vi "AddParametersToCMD.vi"(8 "error in (no error)":errorcluster, 10 "DynamicParameters in":refnum<class "DynamicParameters.lvclass">, 11 "CreateCommand":refnum<k24>) -> (0 "error out":errorcluster, 3 "CreateCommand Out":refnum<k24>)   [LabVIEW 2020, in "ORM_ADONet.lvlib" / "ADOMapper.lvclass"]
uses:
  ADOMapper.lvclass
  System.Data
  <vilib>/Viviota/shared/ORM.lvlibp/ORM/DynamicParameters/DynamicParameters.lvclass
  ADOParameter/ADOParameter.lvclass
  C:/Viviota/Projects/R&D/__OpenSource/VIV_ORM/libraries/npgsql/System.Text.Json.dll
  libraries/npgsql/System.Text.Json.dll
  <userlib>/_OpenG.lib/lvdata/lvdata.llb/openg_variant.lvlib
panel:
  out "error out 5":errorcluster
  out "error out 4":errorcluster
  out "error out 3":errorcluster
  out "error out 2":errorcluster
  out "DbType":i32[](array[ring]) items=["AnsiString"=0, "Binary"=1, "Byte"=2, "Boolean"=3, "Currency"=4, "Date"=5, "DateTime"=6, "Decimal"=7, "Double"=8, "Guid"=9, "Int16"=10, "Int32"=11, "Int64"=12, "Object"=13, "SByte"=14, "Single"=15, "String"=16, "Time"=17, "UInt16"=18, "UInt32"=19, "UInt64"=20, "VarNumeric"=21, "AnsiStringFixedLength"=22, "StringFixedLength"=23, "Xml"=25, "DateTime2"=26, "DateTimeOffset"=27]
  out "Array 2":string[](array[string])
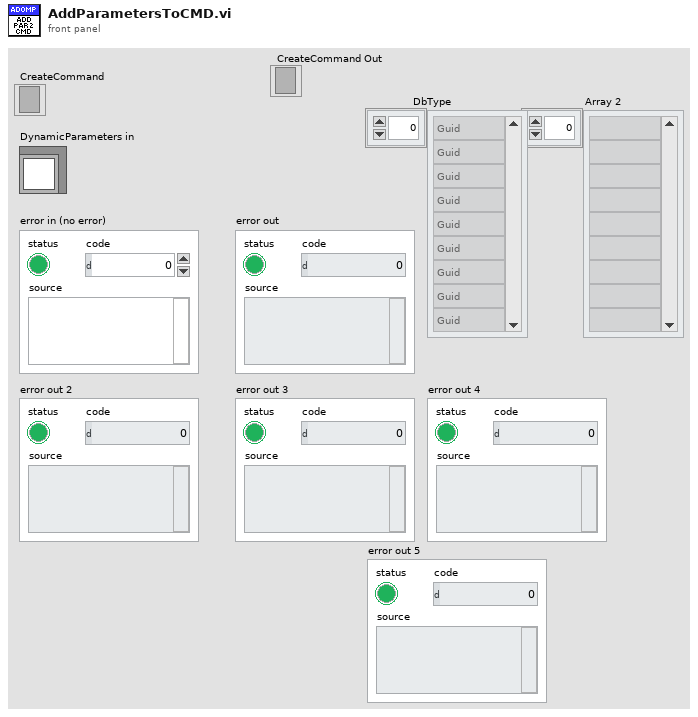
[diagram p1: front panel]
types:
  T1 = cluster{"DbType":i32, "Direction":i32, "Size":i32, "Precision":u8, "Scale":u8}[]
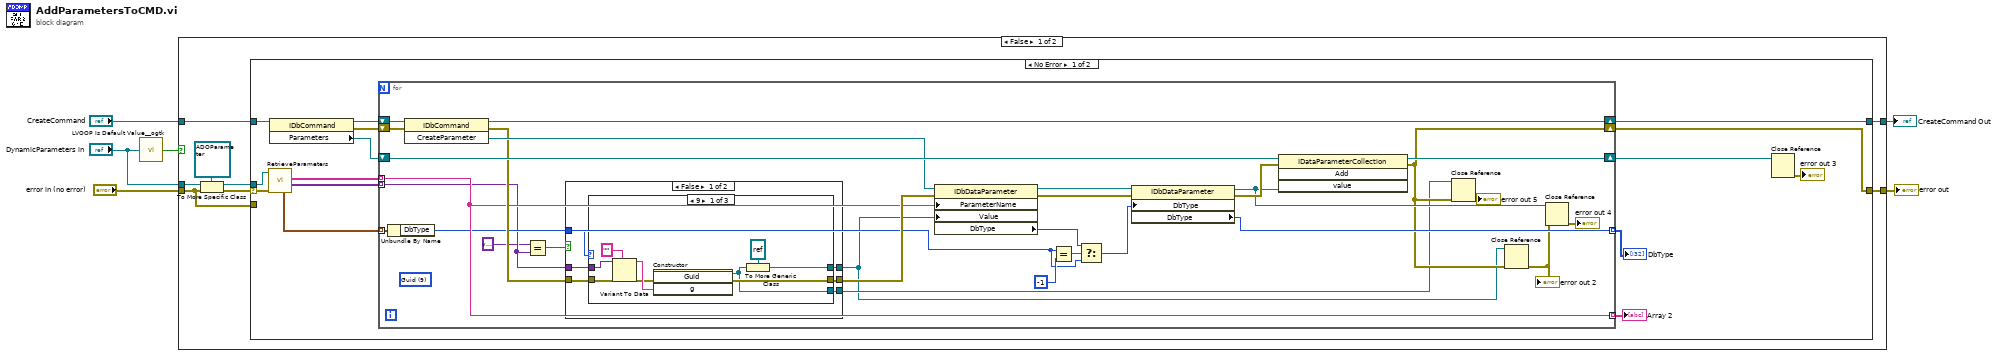
[diagram p0: block diagram]
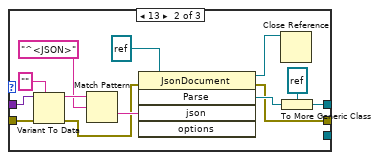
[diagram p2: hidden frame]
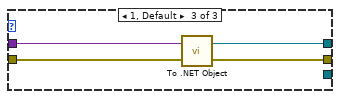
[diagram p3: hidden frame]
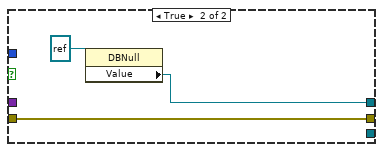
[diagram p4: hidden frame]
diagram:
  n1 = call <userlib>:"LVOOP Is Default Value__ogtk.vi"("Object"="DynamicParameters in") -> ("Is Default Value?"=w3:bool)
  n2 = case shown="False" w3 {
    tunnel: "error in (no error)" -> [w11 w97]
    tunnel: [w7 w97] -> w6
    tunnel: "DynamicParameters in" -> [w13 _]
    tunnel: "CreateCommand" -> [w9 w96]
    tunnel: [w8 w96] -> w1
    frame False {
      n3 = To More Specific Class(target class=refnum<class "ADOParameter.lvclass"> refnum ("ADONet.lvlib:ADOParameter.lvclass"), reference=w13, error in=w11) -> (specific class reference=w10:refnum<class "ADOParameter.lvclass">, error out=w12:errorcluster)
      n4 = case shown="No Error" w12 {
        selector: w12 -> [w29 w94]
        tunnel: w11 -> [_ _]
        tunnel: w10 -> [w28 _]
        tunnel: w9 -> [w27 w95]
        tunnel: [w21 w95] -> w8
        tunnel: [w20 w94] -> w7
        frame No Error {
          n5 = call "RetrieveParameters.vi"("error in (no error)"=w29, "ADOParameter in"=w28) -> ("Values"=w23:variant[], "Names"=w24:string[], "Options"=w18:T1)  [unwired: 5 in, 2 out]
          n6 = property class="IDbCommand"(reference=w27) -> (reference out=w26:refnum<k24>, error out=w22:errorcluster, "Parameters"=w25:refnum<k24>)  [unwired: 1 in]
          n7 = for {
            shift-right: [w51] -> w21
            shift-left: w26 -> [w58]
            shift-right: [w56] -> w15
            shift-left: w25 -> [w57]
            tunnel: w24 -> [w50] mode=indexing
            tunnel: w23 -> [w40] mode=indexing
            shift-right: [w33] -> w20
            shift-left: w22 -> [w52]
            tunnel: [w43] -> w17 mode=indexing
            tunnel: [w50] -> w19 mode=indexing
            tunnel: w18 -> [w42] mode=indexing
            (unwired) 9 items=["AnsiString"=0, "Binary"=1, "Byte"=2, "Boolean"=3, "Currency"=4, "Date"=5, "DateTime"=6, "Decimal"=7, "Double"=8, "Guid"=9, "Int16"=10, "Int32"=11, "Int64"=12, "Object"=13, "SByte"=14, "Single"=15, "String"=16, "Time"=17, "UInt16"=18, "UInt32"=19, "UInt64"=20, "VarNumeric"=21, "AnsiStringFixedLength"=22, "StringFixedLength"=23, "Xml"=25, "DateTime2"=26, "DateTimeOffset"=27] ("DbType")
            n8 = Unbundle By Name(w42) -> ("DbType"=w41:i32)
            n9 = invoke class="IDbCommand" method="CreateParameter"(reference=w58, error in=w52) -> (reference out=w51:refnum<k24>, error out=w54:errorcluster, "CreateParameter"=w55:refnum<k24>)  [unwired: 1 in]
            n10 = Equal?(x=variant, y=w40) -> (x = y?=w37:bool)
            n11 = case shown="False" w37 {
              tunnel: w54 -> [w64 w93]
              tunnel: [w63 w93] -> w53
              tunnel: w41 -> [w62 _]
              tunnel: [w61 w91] -> w30
              tunnel: w40 -> [w60 _]
              tunnel: [w59 _] -> w32
              frame False {
                n12 = case shown="9" w62 {
                  tunnel: [w67 w74 w87] -> w61
                  tunnel: w64 -> [w73 w75 w90]
                  tunnel: [w68 w78 w89] -> w63
                  tunnel: w60 -> [w72 w76 w88]
                  tunnel: [w65 _ _] -> w59
                  frame 9 {
                    n13 = Variant To Data(error in=w73, type="", Variant=w72) -> (data=w70:string, error out=w69:errorcluster)
                    n14 = constructor class="System.Guid" ("Constructor Node")(error in=w69, "g"=w70) -> (reference out=w65:refnum<k24>, error out=w68:errorcluster)  [unwired: 2 in, 2 out]
                    n15 = To More Generic Class(target class=refnum<k24> refnum ("Value"), reference=w65) -> (generic class reference=w67:refnum<k24>)
                  }
                  frame 13 {
                    n16 = Variant To Data(error in=w75, type="", Variant=w76) -> (data=w85:string, error out=w81:errorcluster)
                    n17 = Match Pattern(string=w85, regular expression="^<JSON>") -> (after substring=w82:string)  [unwired: 1 in, 3 out]
                    n18 = invoke class="JsonDocument" method="Parse"(reference=refnum<k24> refnum ("Value"), error in=w81, "json"=w82) -> (reference out=w79:refnum<k24>, error out=w78:errorcluster, "Parse"=w80:refnum<k24>)  [unwired: 2 in, 2 out]
                    n19 = Close Reference(reference=w79) -> ()  [unwired: 1 in, 1 out]
                    n20 = To More Generic Class(target class=refnum<k24> refnum ("Value"), reference=w80) -> (generic class reference=w74:refnum<k24>)
                  }
                  frame 1, Default {
                    n21 = call <vilib>:"To .NET Object.vi"("error in (no error)"=w90, "anything"=w88) -> ("error out"=w89:errorcluster, ".NET object"=w87:refnum<k24>)
                  }
                }
              }
              frame True {
                n22 = property class="DBNull"(reference=refnum<k24> refnum ("CreateParameter")) -> ("Value"=w91:refnum<k24>)  [unwired: 1 in, 2 out]
              }
            }
            n23 = property class="IDbDataParameter"(reference=w55, error in=w53, "ParameterName"=w50, "Value"=w30) -> (reference out=w49:refnum<k24>, error out=w47:errorcluster, "DbType"=w38:i32)
            n24 = Equal?(x=w41, y=-1) -> (x = y?=w45:bool)
            n25 = Select(t=w38, s=w45, f=w41) -> (s? t:f=w46:i32)
            n26 = property class="IDbDataParameter"(reference=w49, error in=w47, "DbType"=w46) -> (reference out=w36:refnum<k24>, error out=w48:errorcluster, "DbType"=w43:i32)
            n27 = invoke class="IDataParameterCollection" method="Add"(reference=w57, error in=w48, "value"=w36) -> (reference out=w56:refnum<k24>, error out=w33:errorcluster)  [unwired: 1 in, 2 out]
            n28 = Close Reference(reference=w32, error in (no error)=w33) -> (error out=→"error out 5":errorcluster)
            n29 = Close Reference(reference=w30, error in (no error)=w33) -> (error out=w35:errorcluster)
            "error out 2" <- w35
            n30 = Close Reference(reference=w36, error in (no error)=w35) -> (error out=→"error out 4":errorcluster)
          }
          "Array 2" <- w19
          "DbType" <- w17
          n31 = Close Reference(reference=w15) -> (error out=→"error out 3":errorcluster)  [unwired: 1 in]
        }
        frame Error {
        }
      }
    }
    frame True {
    }
  }
  "error out" <- w6
  "CreateCommand Out" <- w1
